vi "Conversion_DBL-2INT.vi"(4 "error in":errorcluster, 5 "Integer LOW":u32, 6 "Integer HIGH":u32, 7 "Double":dbl=3.140000104904175 format="%.2f") -> (0 "error out":errorcluster, 1 "Double":dbl, 2 "Integer LOW":u32, 3 "Integer HIGH":u32)   [LabVIEW 2014]
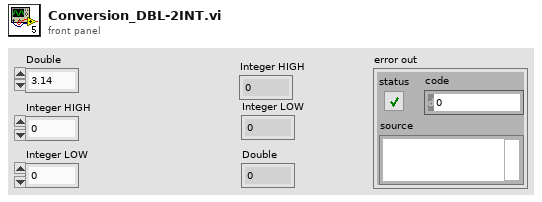
[diagram p1: front panel]
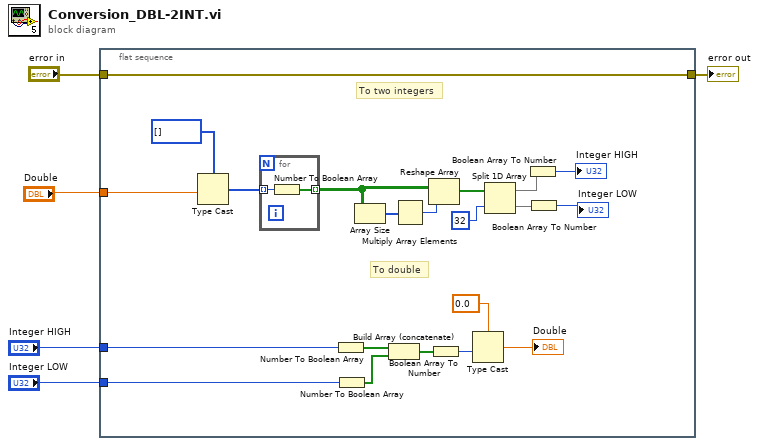
[diagram p0: block diagram]
diagram:
  n1 = flat-sequence {
    tunnel: "Double" -> [w9]
    tunnel: "Integer HIGH" -> [w8]
    tunnel: "Integer LOW" -> [w7]
    tunnel: "error in" -> [w6]
    tunnel: [w6] -> w1
    frame #0 {
      # "To double"
      # "To two integers"
      n2 = Type Cast(type=u32[] [], x=w9) -> (*(type *) &x=w23:u32[])
      n3 = for {
        tunnel: w23 -> [w28] mode=indexing
        tunnel: [w27] -> w26 mode=indexing
        n4 = Number To Boolean Array(number=w28) -> (Boolean array=w27:bool[])
      }
      n5 = Number To Boolean Array(number=w8) -> (Boolean array=w12:bool[])
      n6 = Number To Boolean Array(number=w7) -> (Boolean array=w11:bool[])
      n7 = Array Size(array=w26) -> (size(s)=w22:i32[])
      n8 = Build Array (concatenate)(w12, w11) -> (w10:bool[])
      n9 = Multiply Array Elements(1:w22) -> (0:w25:i32)
      n10 = Reshape Array(w26, w25) -> (w20:bool[])
      n11 = Boolean Array To Number(Boolean array=w10) -> (number=w15:u32)
      n12 = Type Cast(type=0.0 ("Numeric 2"), x=w15) -> (*(type *) &x=→"Double":dbl)
      n13 = Split 1D Array(array=w20, index=u32 32) -> (first subarray=w19:bool[], second subarray=w18:bool[])
      n14 = Boolean Array To Number(Boolean array=w19) -> (number=→"Integer HIGH":u32)
      n15 = Boolean Array To Number(Boolean array=w18) -> (number=→"Integer LOW":u32)
    }
  }
  "error out" <- w1
